vi "TestStand_Control ( Switch_View ).vi"(8 "error in":errorcluster, 10 "View":string, 11 "TestStand UI Data":T1) -> (0 "error out":errorcluster)   [LabVIEW 2018, in "TestStand_Control.lvlib"]
uses:
  Module_Controls/TestStand UI Data.ctl
  TestStand_Control.lvlib
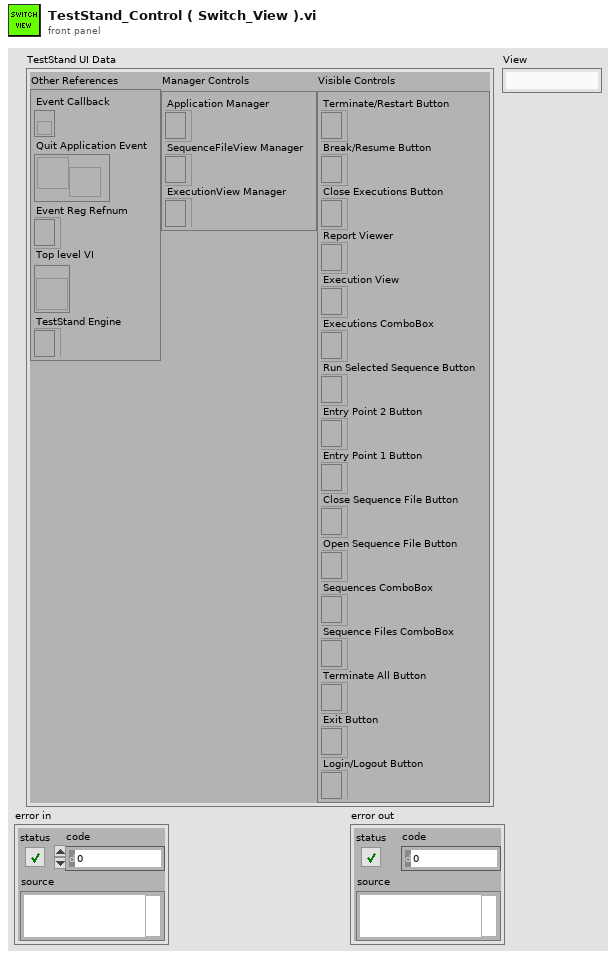
[diagram p1: front panel]
types:
  T1 = typedef "TestStand_Control.lvlib/TestStand UI Data.ctl" = cluster{"Other References":cluster{"Event Callback":refnum<k27>, "Quit Application Event":refnum<user-event>, "Event Reg Refnum":refnum<event-registration>, "Top level VI":refnum<vi>, "TestStand Engine":refnum<k7>}, "Manager Controls":cluster{"Application Manager":refnum<k7>, "SequenceFileView Manager":refnum<k7>, "ExecutionView Manager":refnum<k7>}, "Visible Controls":cluster{"Terminate/Restart Button":refnum<k7>, "Break/Resume Button":refnum<k7>, "Close Executions Button":refnum<k7>, "Report Viewer":refnum<k7>, "Execution View":refnum<k7>, "Executions ComboBox":refnum<k7>, "Run Selected Sequence Button":refnum<k7>, "Entry Point 2 Button":refnum<k7>, "Entry Point 1 Button":refnum<k7>, "Close Sequence File Button":refnum<k7>, "Open Sequence File Button":refnum<k7>, "Sequences ComboBox":refnum<k7>, "Sequence Files ComboBox":refnum<k7>, "Terminate All Button":refnum<k7>, "Exit Button":refnum<k7>, "Login/Logout Button":refnum<k7>}}
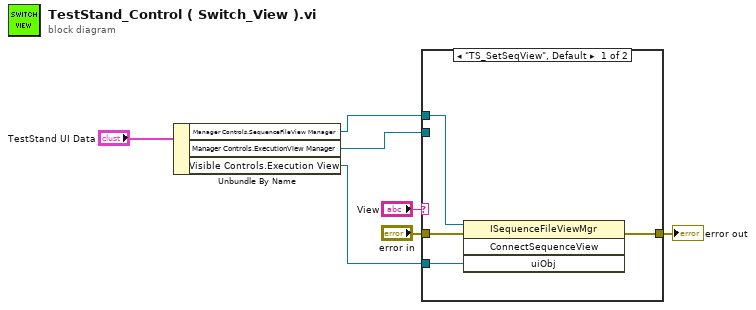
[diagram p0: block diagram]
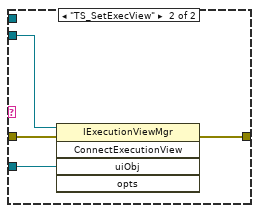
[diagram p2: hidden frame]
diagram:
  n1 = Unbundle By Name("TestStand UI Data") -> ("Manager Controls.SequenceFileView Manager"=w6:refnum<k7>, "Manager Controls.ExecutionView Manager"=w5:refnum<k7>, "Visible Controls.Execution View"=w4:refnum<k7>)
  n2 = case shown="\"TS_SetSeqView\", Default" "View" {
    tunnel: "error in" -> [w11 w15]
    tunnel: [w10 w14] -> w2
    tunnel: w4 -> [w9 w13]
    tunnel: w5 -> [_ w12]
    tunnel: w6 -> [w8 _]
    frame "TS_SetSeqView", Default {
      n3 = invoke class="ISequenceFileViewMgr" method="ConnectSequenceView"(reference=w8, error in=w11, "uiObj"=w9) -> (error out=w10:errorcluster)  [unwired: 1 in, 3 out]
    }
    frame "TS_SetExecView" {
      n4 = invoke class="IExecutionViewMgr" method="ConnectExecutionView"(reference=w12, error in=w15, "uiObj"=w13) -> (error out=w14:errorcluster)  [unwired: 2 in, 4 out]
    }
  }
  "error out" <- w2
